vi "Library Error Code.vi"(11 "error":errorcluster) -> (4 "error code enum":T1, 8 "error code":i32, 15 "dup error":errorcluster)   [LabVIEW 2012]
doc: "Takes an error cluster and returns the error code as well as a corresponding enum for the most popular error causes. The latter allows error code dependent stuff to be selected by wiring the enum into a case structure. If no error is set, this VI returns the \"No error\" enum value and 0 code irrespective of the code.\n\nThis VI is able to retrieve the error code from explained errors. This allows error code dependent stuff to be done somewhere downstream from the error source without having to postpone explaning the error."
uses:
  typedefs/et_Library Error Code Enum.ctl
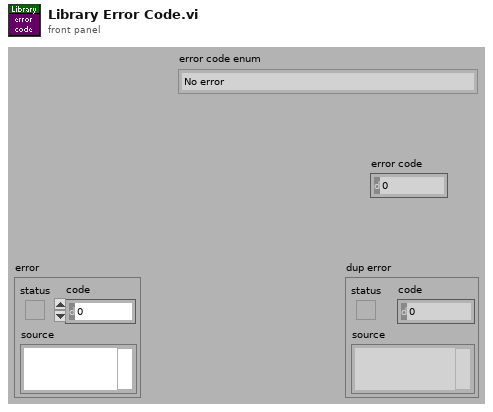
[diagram p1: front panel]
types:
  T1 = typedef "et_Library Error Code Enum.ctl" = enum32{"No error", "Argument error", "Memory is full", "Out of zone", "End of file", "File already open", "Generic file I/O error", "File not found", "File permission error", "Disk is full", "Duplicate path", "Too many files open", "System feature not enabled", "Resource file not found", "Cannot add resource", "Resource not found", "Image not found", "Image memory error", "Pen does not exist", "Config type invalid", "Config token not found", "Config parse error", "Config memory error", "Bad external code format", "Bad external code offset", "External code not present", "Null window", "Destroy window error", "Null menu", "Print aborted", "Bad print record", "Print driver error", "Windows error during printing", "Memory error during printing", "Print dialog error", "Generic print error", "Invalid device refnum", "Device not found", "Device parameter error", "Device unit error", "Cannot open device", "Device call aborted", "Generic error", "Cancelled by user", "Object ID too low", "Object ID too high", "Object not in heap", "Unknown heap", "Unknown object (invalid DefProc)", "Unknown object (DefProc not in table)", "Message out of range", "Invalid (null) method", "Unknown message", "Manager call not supported", "Bad address", "Network operation in progress", "Network operation timed out", "Connection is busy", "Network attribute not supported", "Network error", "Address in use", "System out of memory", "Connection aborted", "Connection refused", "Not connected", "Already connected", "Connection closed", "Initialization error (interapplication manager)", "Bad occurrence", "Wait on unbound occurrence handler", "Occurrence queue overflow", "Datalog type conflict", "Unused", "Unrecognized type (interapplication manager)", "Memory corrupt", "Failed to make temporary DLL", "Old CIN version", "Drag socket not found", "Failed to load drop-object", "Failed to register OLE object", "Failed to release OLE object", "Format specifier type mismatch", "Unknown format specifier", "Too few format specifiers", "Too many format specifiers", "Scan failed", "Newer CIN version", "Error converting to variant", "Runtime menu error", "Password tampered", "Variant attribute not found", "Incompatible variant data type", "Event data is not available", "Event Store is not present", "Occurrence is not found", "Event Queue is not created", "Event info is not available in the type library", "Refnum passed is NULL", "Error retrieving Class GUID", "Error retrieving CoClass GUID", "Error retrieving TypeLib GUID.", "Bad built application magic bytes.", "Specific driver is different from the specific driver associated with the Logical Name.", "There is no session opened to the class driver.", "Max Error", "MAX - Error with config objects", "MAX - Error loading configuration", "MAX - Group not supported", "Singlecast connections can not send to multicast addresses.", "Multicast connections can not send to singlecast addresses.", "Specified IP address not in multicast address range.", "Attempt to write to read-only multicast connection.", "Attempt to read from write-only multicast connection.", "The buffer used to receive a datagram was smaller than the datagram itself", "Error code not enumerated"}
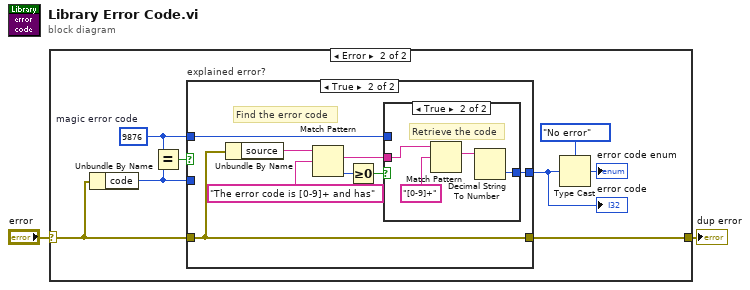
[diagram p0: block diagram]
diagram:
  n1 = case shown="Error" "error" {
    selector: "error" -> [w3 w11]
    tunnel: [w3 w7] -> w1
    frame No Error {
    }
    frame Error {
      w4 = 9876  # magic error code
      n2 = Unbundle By Name(w11) -> ("code"=w5:i32)
      n3 = Equal?(x=w4, y=w5) -> (x = y?=w6:bool)
      n4 = case "explained error?" shown="True" w6 {
        tunnel: w5 -> [w13 _]
        tunnel: w11 -> [w12 w15]
        tunnel: [w13 w17] -> w8
        tunnel: [w12 w15] -> w7
        tunnel: w4 -> [_ w16]
        frame False {
        }
        frame True {
          # "Find the error code"
          n5 = Unbundle By Name(w15) -> ("source"=w14:string)
          n6 = Match Pattern(string=w14, regular expression="The error code is [0-9]+ and has") -> (match substring=w21:string, offset past match=w19:i32)  [unwired: 1 in, 2 out]
          n7 = Greater Or Equal To 0?(x=w19) -> (x >= 0?=w18:bool)
          n8 = case shown="True" w18 {
            tunnel: w21 -> [_ w25]
            tunnel: [w22 w23] -> w17
            tunnel: w16 -> [w22 _]
            frame False {
            }
            frame True {
              # "Retrieve the code"
              n9 = Match Pattern(string=w25, regular expression="[0-9]+") -> (match substring=w26:string)  [unwired: 1 in, 3 out]
              n10 = Decimal String To Number(string=w26) -> (number=w23:i32)  [unwired: 2 in, 1 out]
            }
          }
        }
      }
      "error code" <- w8
      n11 = Type Cast(type=et_Library_Error_Code_Enum."No error" ("errors"), x=w8) -> (*(type *) &x=→"error code enum":T1)
    }
  }
  "dup error" <- w1
